vi "Init Constructor Parser.vi"(10 "Token List":T1[](array[typedef]), 11 "Input":string) -> (3 "Constructor String Parser":T3={"Input"="", "Token List"=[], "Result"={"protocol"="", "username"="", "password"="", "hostname"="", "port"="", "pathname"="", "search"="", "hash"=""}, "Component Start"=0, "Token Index"=0, "Token Increment"=1, "Group Depth"=0, "Hostname IPv6 Bracket Depth"=0, "Protocol Matches Special Scheme"=FALSE, "State"=enum."init", "List Length"=0})   [LabVIEW 2020, in "Stream.lvlib" / "URLPattern.lvclass"]
uses:
  URLPattern.lvclass
  Token Type.ctl
  Token.ctl
  URL Pattern Init.ctl
  Parser State.ctl
  Constructor String Parser.ctl
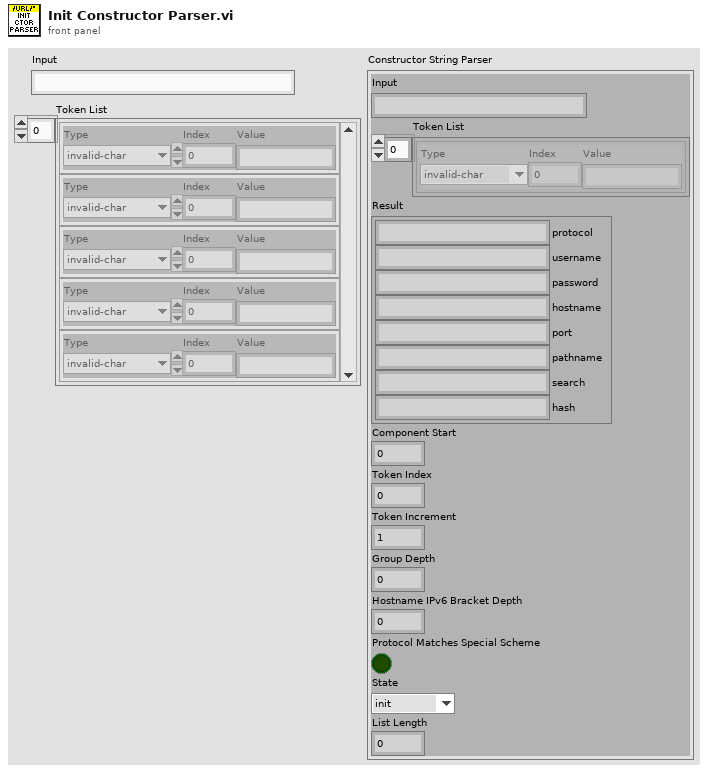
[diagram p1: front panel]
types:
  T1 = typedef "Stream.lvlib/URLPattern.lvclass/Token.ctl" = cluster{"Type":T2, "Index":i32, "Value":string}
  T2 = typedef "Stream.lvlib/URLPattern.lvclass/Token Type.ctl" = enum16{"invalid-char", "open", "close", "regexp", "name", "char", "escaped-char", "other-modifier", "asterisk", "end"}
  T3 = typedef "Stream.lvlib/URLPattern.lvclass/Constructor String Parser.ctl" = cluster{"Input":string, "Token List":T1[], "Result":T4, "Component Start":i32, "Token Index":i32, "Token Increment":i32, "Group Depth":i32, "Hostname IPv6 Bracket Depth":i32, "Protocol Matches Special Scheme":bool, "State":T5, "List Length":i32}
  T4 = typedef "Stream.lvlib/URLPattern.lvclass/URL Pattern Init.ctl" = cluster{"protocol":string, "username":string, "password":string, "hostname":string, "port":string, "pathname":string, "search":string, "hash":string}
  T5 = typedef "Stream.lvlib/URLPattern.lvclass/Parser State.ctl" = enum16{"init", "protocol", "authority", "username", "password", "hostname", "port", "pathname", "search", "hash", "done"}
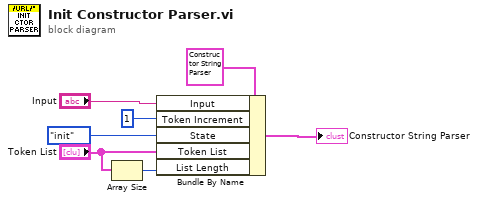
[diagram p0: block diagram]
diagram:
  n1 = Array Size(array="Token List") -> (size(s)=w1:i32)
  n2 = Bundle By Name(cluster=T3 {"Input"="", "Token List"=[], "Result"={"protocol"="", "username"="", "password"="", "hostname"="", "port"="", "pathname"="", "search"="", "hash"=""}, "Component Start"=0, "Token Index"=0, "Token Increment"=0, "Group Depth"=0, "Hostname IPv6 Bracket Depth"=0, "Protocol Matches Special Scheme"=FALSE, "State"=enum."init", "List Length"=0} ("Constructor String Parser"), "Input"="Input", "Token Increment"=1, "State"=Parser_State."init", "Token List"="Token List", "List Length"=w1) -> (→"Constructor String Parser":T3)
